vi "OE2031&OE2041_Configure Input Filter.vi"(7 "OE2041_Configure Input Filter":T1 {"Input Impedance" items=["50Ω", "10MΩ"]; "Input Coupling" items=["AC", "DC"]; "Input Shield Grounding" items=["Float", "Ground"]; "Input Source" items=["A", "B"]}, 8 "Error in (no error)":errorcluster caption="error out（no error）", 9 "Remote Mode":u16(ring) items=["USB", "RS232", "GPIB", "Ethernet"], 10 "Connection ID in":refnum<k5>, 11 "VISA resource name":refnum<visa-resource-name>) -> (0 "Error out":errorcluster caption="error out", 1 "Output String":string, 2 "Connection ID out":refnum<k5>, 3 "VISA resource  out":refnum<visa-resource-name>)   [LabVIEW 2011]
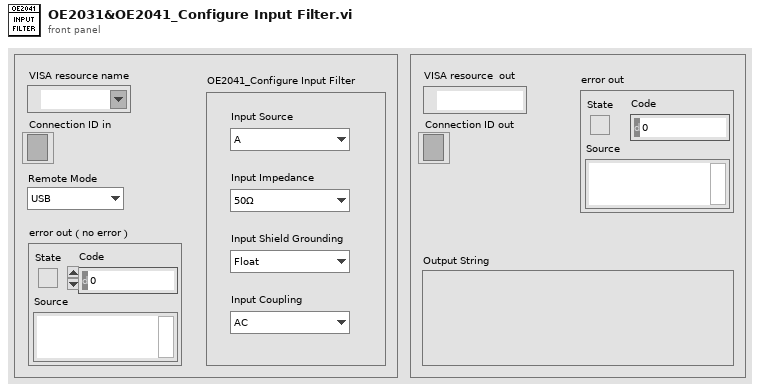
[diagram p1: front panel]
types:
  T1 = cluster{"Input Source":u16, "Input Shield Grounding ":u16, "Input Coupling ":u16, "Input Impedance ":u16}
  T2 = enum16{"ISRC", "IGND", "ICPL", "ILIN", "PHAS", "FMOD", "RSLP", "FREQ", "SWPT", "SLLM", "SULM", "SSLL", "SSLG", "STLM", "SWRM", "IRNG", "SENS", "RMOD", "OFLT", "OFSL", "SYNC", "DMOD", "HARM", "DARB", "SWVT", "SLVL", "SVLL", "SVUL", "SVSL", "SVSG", "SVTM", "SVRM", "RALL", "SNAP", "OUTP", "OAUX", "COUT", "CAUX", "COFP", "CEXP", "FPOP", "OEXP", "*IDN", "*RST", "OVLD", "INOV", "GNOV", "*PLL", "SSET", "RSET", "AGAN", "APHS", "ARSV", "ASCL", "EQCD", "EQCS", "SPED", "SRAT", "SLEN", "SSLE", "STRG", "SPRM", "STRD", "PAUS", "REST", "SPTS", "TRCA", "TEMP", "RSTU", "IHNZ", "DEQU", "SADD", "ARNG", "CSPE", "ISRCD", "IGNDD", "ICPLD", "ILIND", "PHASD", "FMODD", "RSLPD", "FREQD", "SWPTD", "SLLMD", "SULMD", "SSLLD", "SSLGD", "STLMD", "SWRMD", "SENSD", "RMODD", "OFLTD", "OFSLD", "SYNCD", "HARMD", "EQCDD", "EQCSD", "SNAPD", "OUTPD", "SWVTD", "SLVLD", "SVLLD", "SVULD", "SVSLD", "SVSGD", "SVTMD", "SVRMD", "SVDCD", "ARSVD", "AGAND", "APHSD", "ASCLD", "FPOPD", "CAUXD", "OEXPD", "SPEDD", "SRATD", "SLEND", "SSLED", "STRGD", "SPRMD", "STRDD", "PAUSD", "RESTD", "SPTSD", "TRCAD", "*IDND", "*RSTD", "INOVD", "GNOVD", "*PLLD", "SSETD", "RSETD"}
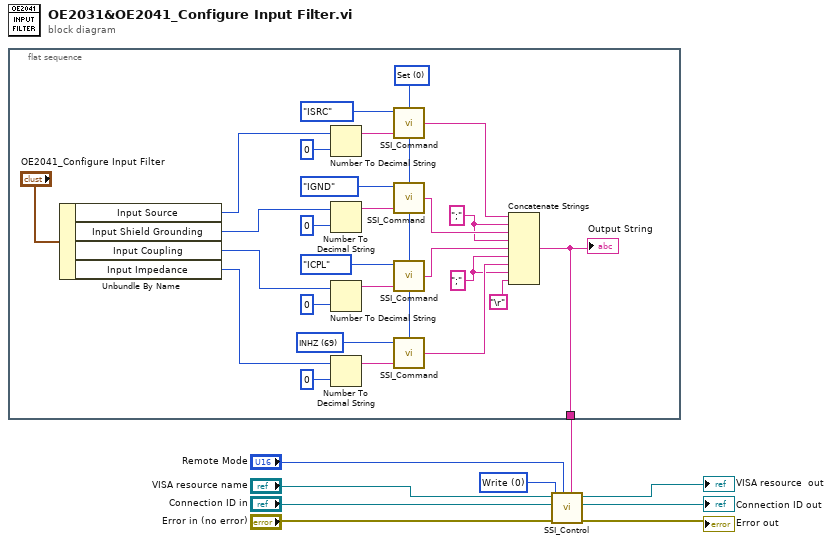
[diagram p0: block diagram]
diagram:
  w7 = u16 0 items=["Write", "Read"] ("Control")
  n1 = flat-sequence {
    tunnel: [w11] -> w1
    frame #0 {
      w10 = u16 69 items=["ISRC", "IGND", "ICPL", "ILIN", "PHAS", "FMOD", "RSLP", "FREQ", "SWPT", "SLLM", "SULM", "SSLL", "SSLG", "STLM", "SWRM", "IRNG", "SENS", "RMOD", "OFLT", "OFSL", "SYNC", "DMOD", "HARM", "DARB", "SWVT", "SLVL", "SVLL", "SVUL", "SVSL", "SVSG", "SVTM", "SVRM", "RALL", "SNAP", "OUTP", "OAUX", "COUT", "CAUX", "COFP", "CEXP", "FPOP", "OEXP", "*IDN", "*RST", "OVLD", "INOV", "GNOV", "*PLL", "SSET", "RSET", "AGAN", "APHS", "ARSV", "ASCL", "EQCD", "EQCS", "SPED", "SRAT", "SLEN", "SSLE", "STRG", "SPRM", "STRD", "PAUS", "RSET", "SPTS", "TRCA", "TEMP", "RSTU", "INHZ", "DEQU", "SADD", "ARNG", "CSPE", "ISRCD", "IGNDD", "ICPLD", "ILIND", "PHASD", "FMODD", "RSLPD", "FREQD", "SWPTD", "SLLMD", "SULMD", "SSLLD", "SSLGD", "STLMD", "SWRMD", "SENSD", "RMODD", "OFLTD", "OFSLD", "SYNCD", "HARMD", "EQCDD", "EQCSD", "SNAPD", "OUTPD", "SWVTD", "SLVLD", "SVLLD", "SVULD", "SVSLD", "SVSGD", "SVTMD", "SVRMD", "SVDCD", "ARSVD", "AGAND", "APHSD", "ASCLD", "FPOPD", "CAUXD", "OEXPD", "SPEDD", "SRATD", "SLEND", "SSLED", "STRGD", "SPRMD", "STRDD", "PAUSD", "RESTD", "SPTSD", "TRCAD", "*IDND", "*RSTD", "INOVD", "GNOVD", "*PLLD", "SSETD", "RSETD", "RALLD"] ("Command Type")
      w13 = ";" ("字符串")
      w14 = ";" ("字符串")
      w30 = u16 0 items=["Set", "Query"] ("Opera")
      n2 = Unbundle By Name("OE2041_Configure Input Filter") -> ("Input Source"=w34:u16, "Input Shield Grounding"=w33:u16, "Input Coupling"=w32:u16, "Input Impedance"=w31:u16)
      n3 = Number To Decimal String(number=w34, width (-)=i16 0 ("精度(6)")) -> (decimal integer string=w28:string)
      n4 = Number To Decimal String(number=w33, width (-)=i16 0 ("精度(6)")) -> (decimal integer string=w25:string)
      n5 = Number To Decimal String(number=w32, width (-)=i16 0 ("精度(6)")) -> (decimal integer string=w20:string)
      n6 = Number To Decimal String(number=w31, width (-)=i16 0 ("精度(6)")) -> (decimal integer string=w17:string)
      n7 = call "SSI_Command.vi"("Opera"=w30, "Paramter"=w28, "Command Type"=T2."ISRC") -> ("Output string"=w23:string)  [unwired: 1 in]
      n8 = call "SSI_Command.vi"("Opera"=w30, "Paramter"=w25, "Command Type"=T2."IGND") -> ("Output string"=w22:string)  [unwired: 1 in]
      n9 = call "SSI_Command.vi"("Opera"=w30, "Paramter"=w20, "Command Type"=T2."ICPL") -> ("Output string"=w15:string)  [unwired: 1 in]
      n10 = call "SSI_Command.vi"("Opera"=w30, "Paramter"=w17, "Command Type"=w10) -> ("Output string"=w16:string)  [unwired: 1 in]
      n11 = Concatenate Strings(w23, w14, w22, w14, w15, w13, w16, w13, "\r") -> (w11:string)
      "Output String" <- w11
    }
  }
  n12 = call "SSI_Control.vi"("Write Buffer"=w1, "Remote Mode"="Remote Mode", "Error in (no error)"="Error in (no error)", "Control"=w7, "Connection ID in"="Connection ID in", "VISA resource name"="VISA resource name") -> ("Error out"=→"Error out":errorcluster, "Connection ID out"=→"Connection ID out":refnum<k5>, "VISA resource  out"=→"VISA resource  out":refnum<visa-resource-name>)  [unwired: 2 in, 1 out]
